vi "Actuator Home Position.vi"() -> ()   [LabVIEW 2012]
panel:
  in  "Actuator Home Position":dbl
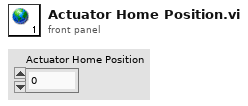
[diagram p1: front panel]
diagram:
